vi "Save Settings to XML.vi"(8 "error in (no error)":errorcluster, 11 "Settings":T1={"Calibration Array"=[], "Hardware Config Cluster"=[], "Trigger Settings"={"Trigger Type"=enum."No Trigger", "Digital Start"={"Source"="", "Digital Start Trigger Edge"=0}, "Digital Pause"={"Source"="APFI0", "Digital Pause Trigger Pause When"=10192}, "Digital Reference"={"Source"="", "Digital Start Trigger Edge"=10280, "Digital Reference Pretrigger Samples"=0}, "Analog Start"={"Source"="", "Analog Slope"=10093, "Analog Start Trigger Hysteresis"=0.0, "Analog Start Trigger Level"=0.0}, "Analog Pause"={"Source"="", "Analog Start Trigger Level"=0.0, "Analog Pause Trigger Pause When"=10093}, "Analog Reference"={"Source"="", "Slope"=10280, "Pretrigger Samples"=0, "Level"=0.0}, "Time Start"={"Select Time\nManually"=FALSE, "When"=timestamp(0 s since 1904-01-01)}}, "Log File Base Path"=path "", "DAQmx Timing Settings"={"rate"=1000.0, "source"="OnboardClock", "sample mode"=10178, "samples per channel"=1000}} {"DAQmx Timing Settings"."sample mode" items=["Finite Samples"=10178, "Continuous Samples"=10123, "Hardware Timed Single Point"=12522]; "DAQmx Timing Settings"."rate" format="%0.2f"; "Trigger Settings"."Time Start"."When" format="%<%x %.3X>T"; "Trigger Settings"."Analog Reference"."Level" format="%0.2f"; "Trigger Settings"."Analog Reference"."Slope" items=["Rising"=10280, "Falling"=10171]; "Trigger Settings"."Analog Pause"."Analog Pause Trigger Pause When" items=["Above Level"=10093, "Below Level"=10107]; "Trigger Settings"."Analog Pause"."Analog Start Trigger Level" format="%0.2f"; "Trigger Settings"."Analog Start"."Analog Start Trigger Level" format="%0.2f"; "Trigger Settings"."Analog Start"."Analog Start Trigger Hysteresis" format="%.2f"; "Trigger Settings"."Analog Start"."Analog Slope" items=["Rising"=10280, "Falling"=10171]; "Trigger Settings"."Digital Reference"."Digital Start Trigger Edge" items=["Rising"=10280, "Falling"=10171]; "Trigger Settings"."Digital Pause"."Digital Pause Trigger Pause When" items=["High"=10192, "Low"=10214]; "Trigger Settings"."Digital Start"."Digital Start Trigger Edge" items=["Rising"=10280, "Falling"=10171]; "Hardware Config Cluster"."Unit" items=["Volts", "From Custom Scale"]}) -> (0 "error out":errorcluster)   [LabVIEW 2020, in "Settings Editor.lvlib"]
doc: "Saves the \"User Specified\" configuration data to an XML file. This is used to remember the users settings between executions.\n_____\nBased on DQMH Project Template 6.0.0.91."
uses:
  Settings Editor.lvlib
  Settings--cluster.ctl
  DAQmx Config--cluster.ctl
  DAQmx Trigger Settings--cluster.ctl
  DAQmx Timing--cluster.ctl
  <vilib>/Utility/xml.llb/Write to XML File(string).vi
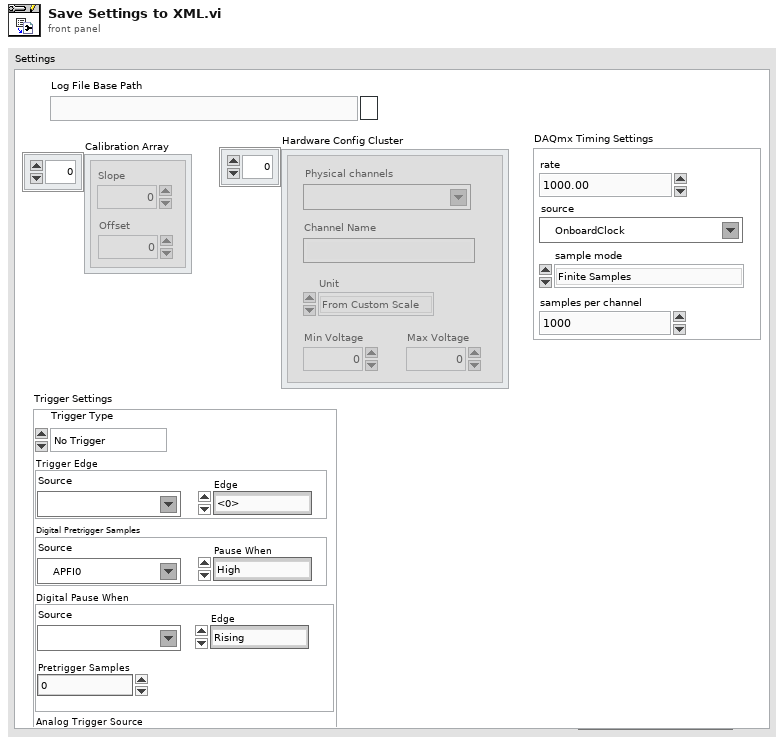
[diagram p1: front panel]
types:
  T1 = typedef "Settings Editor.lvlib/Settings--cluster.ctl" = cluster{"Calibration Array":cluster{"Slope":dbl, "Offset":dbl}[], "Hardware Config Cluster":T2, "Trigger Settings":T3, "Log File Base Path":path, "DAQmx Timing Settings":T4}
  T2 = typedef "Settings Editor.lvlib/DAQmx Config--cluster.ctl" = cluster{"Physical channels":tag, "Channel Name":string, "Unit":i32, "Min Voltage":dbl, "Max Voltage":dbl}[]
  T3 = typedef "Settings Editor.lvlib/DAQmx Trigger Settings--cluster.ctl" = cluster{"Trigger Type":enum32{"No Trigger", "Digital Start", "Digital Pause", "Digital Reference", "Analog Start", "Analog Pause", "Analog Reference", "Time Start"}, "Digital Start":cluster{"Source":tag, "Digital Start Trigger Edge":i32}, "Digital Pause":cluster{"Source":tag, "Digital Pause Trigger Pause When":i32}, "Digital Reference":cluster{"Source":tag, "Digital Start Trigger Edge":i32, "Digital Reference Pretrigger Samples":u32}, "Analog Start":cluster{"Source":string, "Analog Slope":i32, "Analog Start Trigger Hysteresis":dbl, "Analog Start Trigger Level":dbl}, "Analog Pause":cluster{"Source":string, "Analog Start Trigger Level":dbl, "Analog Pause Trigger Pause When":i32}, "Analog Reference":cluster{"Source":string, "Slope":i32, "Pretrigger Samples":u32, "Level":dbl}, "Time Start":cluster{"Select Time\nManually":bool, "When":timestamp}}
  T4 = typedef "Settings Editor.lvlib/DAQmx Timing--cluster.ctl" = cluster{"rate":dbl, "source":tag, "sample mode":i32, "samples per channel":i32}
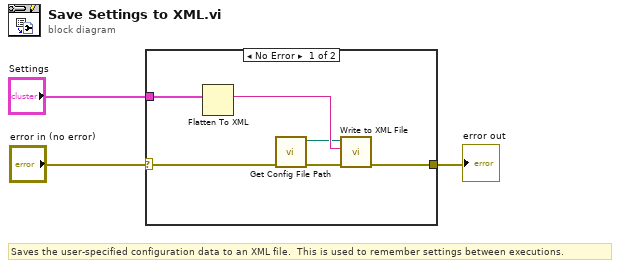
[diagram p0: block diagram]
diagram:
  # "Saves the user-specified configuration data to an XML file.  This is used to remember settings between executions."
  n1 = case shown="No Error" "error in (no error)" {
    selector: "error in (no error)" -> [w5 w10]
    tunnel: [w7 w10] -> w2
    tunnel: "Settings" -> [w9 _]
    frame No Error {
      n2 = Flatten To XML(6:w9) -> (2:w8:string)
      n3 = call "Get Config File Path.vi"("error in (no error)"=w5) -> ("error out"=w4:errorcluster, "XML File Path"=w6:path)  [unwired: 9 in]
      n4 = call-poly <vilib>:"Write to XML File.vi"("error in (no error)"=w4, "XML Input"=w8, "XML File Path"=w6) -> ("error out"=w7:errorcluster)  [unwired: 6 in, 2 out]
    }
    frame Error {
    }
  }
  "error out" <- w2
